vi "S2C_ProcessControl.vi"(8 "Error In":errorcluster, 11 "Action":enum16{"Launch", "Exit"}(ring)) -> (0 "Error Out":errorcluster)   [LabVIEW 2015]
doc: "Sends Viper messages to the TCP Fornax communications connection."
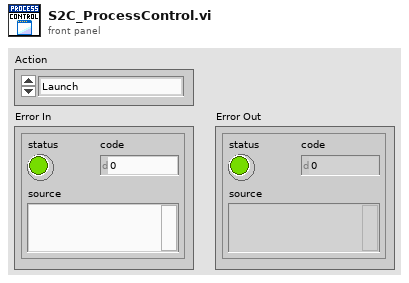
[diagram p1: front panel]
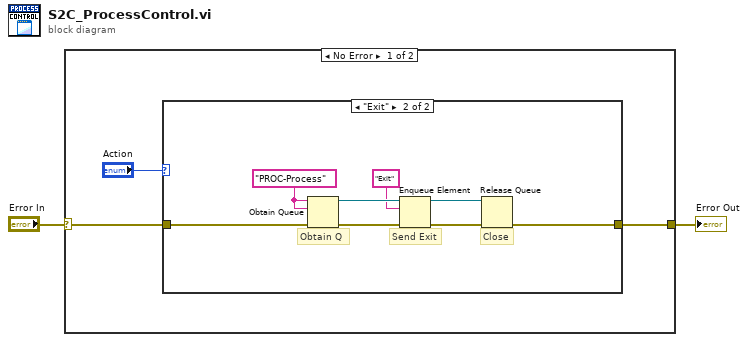
[diagram p0: block diagram]
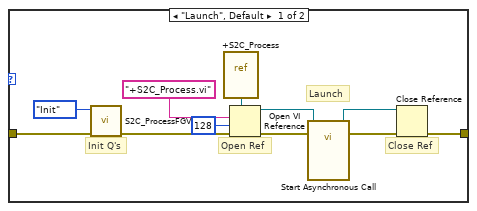
[diagram p2: hidden frame]
diagram:
  n1 = case shown="No Error" "Error In" {
    selector: "Error In" -> [w5 w25]
    tunnel: [w4 w25] -> w1
    frame No Error {
      n2 = case shown="\"Exit\"" "Action" {
        tunnel: w5 -> [w8 w24]
        tunnel: [w9 w18] -> w4
        frame "Launch", Default {
          # "Init Q's"
          # "Close Ref"
          # "Launch"
          # "Open Ref"
          n3 = call "S2C_ProcessFGV.vi"("Error In"=w8, "Action"=enum16{"Init", "Add", "Get"}."Init") -> ("Error Out"=w7:errorcluster)  [unwired: 8 in, 1 out]
          n4 = vi-ref "+S2C_Process.vi"() -> (w14:refnum<vi>)
          n5 = Open VI Reference(type specifier VI Refnum (for type only)=w14, vi path="+S2C_Process.vi", options=128, error in (no error)=w7) -> (vi reference=w12:refnum<vi>, error out=w13:errorcluster)  [unwired: 2 in]
          n6 = call-by-ref "Start Asynchronous Call"(reference=w12, error in=w13) -> (reference out=w16:refnum<vi>, error out=w15:errorcluster)  [unwired: 11 in, 1 out]
          n7 = Close Reference(reference=w16, error in (no error)=w15) -> (error out=w9:errorcluster)
        }
        frame "Exit" {
          w22 = "PROC-Process"
          # "Close"
          # "Obtain Q"
          # "Send Exit"
          n8 = Obtain Queue(name (unnamed)=w22, element data type=w22, error in (no error)=w24) -> (queue out=w21:refnum<queue>, error out=w23:errorcluster)  [unwired: 2 in, 1 out]
          n9 = Enqueue Element(queue=w21, element="Exit", error in (no error)=w23) -> (queue out=w17:refnum<queue>, error out=w19:errorcluster)  [unwired: 1 in, 1 out]
          n10 = Release Queue(queue=w17, error in (no error)=w19) -> (error out=w18:errorcluster)  [unwired: 1 in, 2 out]
        }
      }
    }
    frame Error {
    }
  }
  "Error Out" <- w1
